vi "Average DBL.vi"(6 "Samples to average":i32=1, 10 "Data in":dbl) -> (2 "Averaged data out":dbl)   [LabVIEW 2011]
doc: "This VI averages data over a variable number of samples."
uses:
  <vilib>/Analysis/NI_AALBase.lvlib
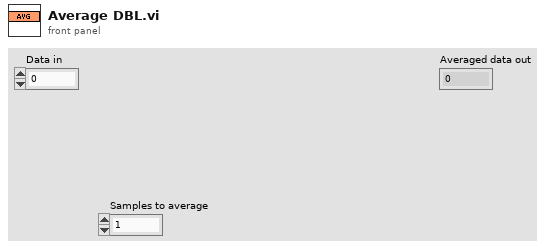
[diagram p1: front panel]
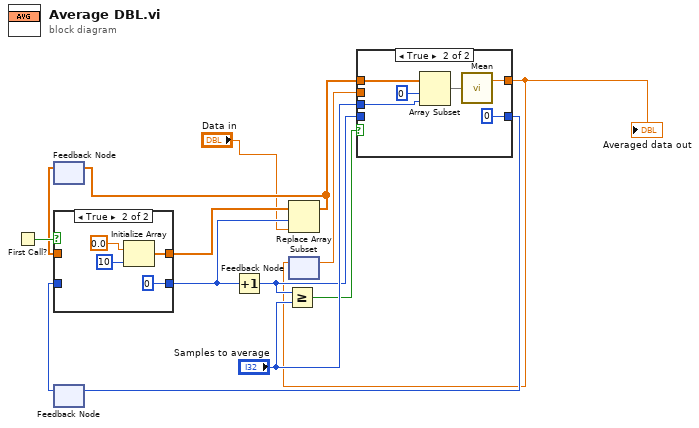
[diagram p0: block diagram]
diagram:
  n1 = First Call?() -> (First Call?: T/F=w13:bool)
  n2 = feedback #1() -> (w11:dbl[])  [unwired: 1 in]
  n3 = feedback #2() -> (w9:i32)  [unwired: 1 in]
  n4 = case shown="True" w13 {
    tunnel: [w15 w17] -> w12
    tunnel: w11 -> [w15 _]
    tunnel: [w14 0 ("index")] -> w10
    tunnel: w9 -> [w14 _]
    frame False {
    }
    frame True {
      n5 = Initialize Array(0.0 ("element"), 10 ("dimension size")) -> (w17:dbl[])
    }
  }
  n6 = Increment(x=w10) -> (x+1=w4:i32)
  n7 = Greater Or Equal?(x=w4, y="Samples to average") -> (x >= y?=w6:bool)
  n8 = Replace Array Subset(array=w12, new element="Data in", index=w10) -> (w8:dbl[])
  n9 = feedback-in #1(w8) -> ()
  n10 = feedback #3() -> (w3:dbl)  [unwired: 1 in]
  n11 = case shown="True" w6 {
    tunnel: w8 -> [_ w27]
    tunnel: "Samples to average" -> [_ w25]
    tunnel: [w21 0 ("t")] -> w5
    tunnel: w4 -> [w21 _]
    tunnel: [w20 w22] -> w2
    tunnel: w3 -> [w20 _]
    frame False {
    }
    frame True {
      n12 = Array Subset(array=w27, index=0, length=w25) -> (w24:dbl[])
      n13 = call <vilib>:"Mean.vi"("X"=w24) -> ("mean"=w22:dbl)  [unwired: 1 out]
    }
  }
  "Averaged data out" <- w2
  n14 = feedback-in #2(w5) -> ()
  n15 = feedback-in #3(w2) -> ()
